vi "Create Tree Item For Add.vi"(8 "Child Only? (true)":bool=TRUE, 9 "Child Text":string, 10 "Left Cell String":string, 11 "Child Tag in":string) -> (1 "Item":T1, 3 "Child Tag out":string)   [LabVIEW 2020, in "Output Sequencer.lvlib" / "Settings UI.lvclass"]
uses:
  Settings UI.lvclass
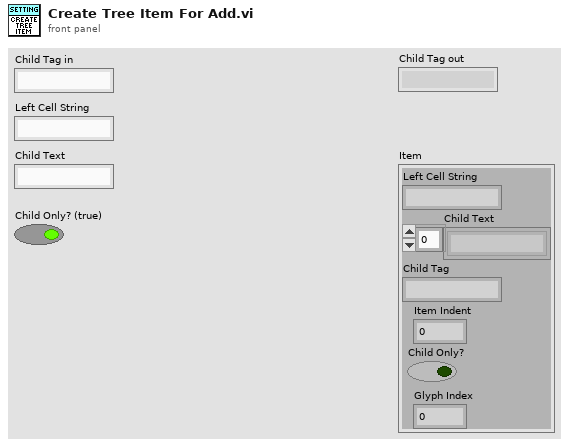
[diagram p1: front panel]
types:
  T1 = cluster{"Left Cell String":string, "Child Text":string[], "Child Tag":string, "Item Indent":i32, "Child Only?":bool, "Glyph Index":i32}
  T2 = typedef "Output Sequencer.lvlib/Settings UI.lvclass/Tree Item Settings.ctl" = cluster{"Tree Label":string, "Indent Level":i32, "Data Type":T3, "Numeric Range":cluster{"Min":dbl, "Max":dbl, "Inc":dbl}, "Allowed Values":string[], "Default Value":string, "Description":string}
  T3 = typedef "Output Sequencer.lvlib/Settings UI.lvclass/Data Type.ctl" = i16
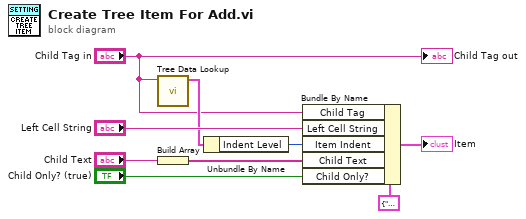
[diagram p0: block diagram]
diagram:
  n1 = call "Tree Data Lookup.vi"("Tag in"="Child Tag in") -> ("Tree Data"=w4:T2)  [unwired: 5 in, 5 out]
  n2 = Build Array("Child Text") -> (w6:string[])
  n3 = Unbundle By Name(w4) -> ("Indent Level"=w3:i32)
  n4 = Bundle By Name(cluster=T1 {"Left Cell String"="", "Child Text"=[], "Child Tag"="", "Item Indent"=0, "Child Only?"=FALSE, "Glyph Index"=0} ("Item"), "Child Tag"="Child Tag in", "Left Cell String"="Left Cell String", "Item Indent"=w3, "Child Text"=w6, "Child Only?"="Child Only? (true)") -> (→"Item":T1)
  "Child Tag out" <- "Child Tag in"
